vi "test - array in seperated but same session.vi"(8 "error in (no error)":errorcluster, 11 "TestCase in":refnum<class "labview-config-library.lvclass">) -> (0 "error out":errorcluster, 3 "TestCase out":refnum<class "labview-config-library.lvclass">)   [LabVIEW 2017, in "labview-config-library.lvclass"]
uses:
  labview-config-library.lvclass
  <vilib>/addons/_JKI Toolkits/VI Tester/TestCase.llb/TestCase.lvclass
  INI-Static-Variable-Support/LabVIEW-Config/LabVIEW-Config.lvclass
  INI-Static-Variable-Support/LabVIEW-Config/Read Array Key (Raw).vi
  C:/Program Files (x86)/National Instruments/LabVIEW 2017/vi.lib/addons/_JKI Toolkits/VI Tester/TestCase.llb/TestCase.lvclass
panel:
  out "appended array":bool[](array[boolean])
  out "text":string
  in  "Tab Control":enum32{"Page 1", "Page 2", "Page 3"}(tab)
  out "Section Names":string[](array[string])
  out "Key Names":string[](array[string])
  out "Array":string[](array[string])
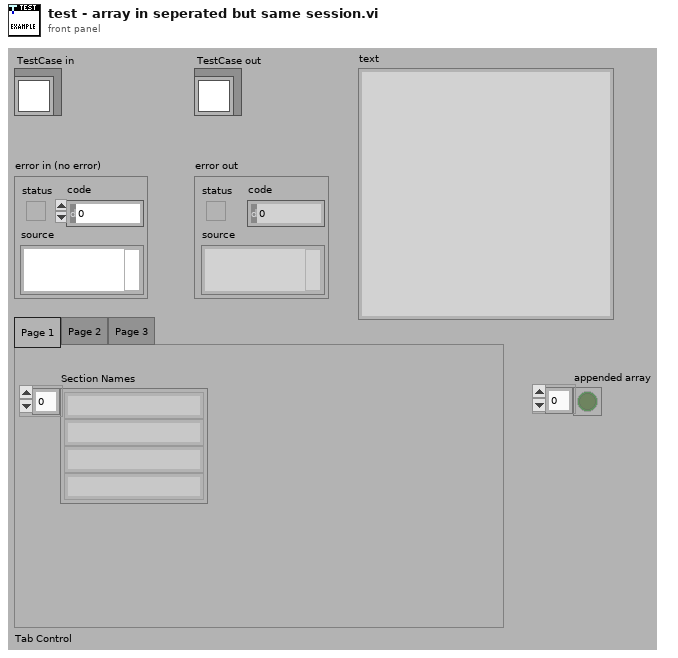
[diagram p1: front panel]
types:
  T1 = typedef "LabVIEW-Config.lvlib/LabVIEW-Config.lvclass/Config.ctl" = cluster{"Path":path, "Lines":string[], "Tokens":T2[], "Modified?":bool, "Cache":cluster{"Valid?":bool, "Key Information":T3[]}}
  T2 = typedef "LabVIEW-Config.lvlib/LabVIEW-Config.lvclass/LineToken.ctl" = enum8{"comment", "section", "key", "more"}
  T3 = typedef "LabVIEW-Config.lvlib/LabVIEW-Config.lvclass/KeyInfo.ctl" = cluster{"Key Indexes":cluster{"Indexes":i32[]}[], "Session Found?":bool, "Key found?":bool, "Session Index":i32}
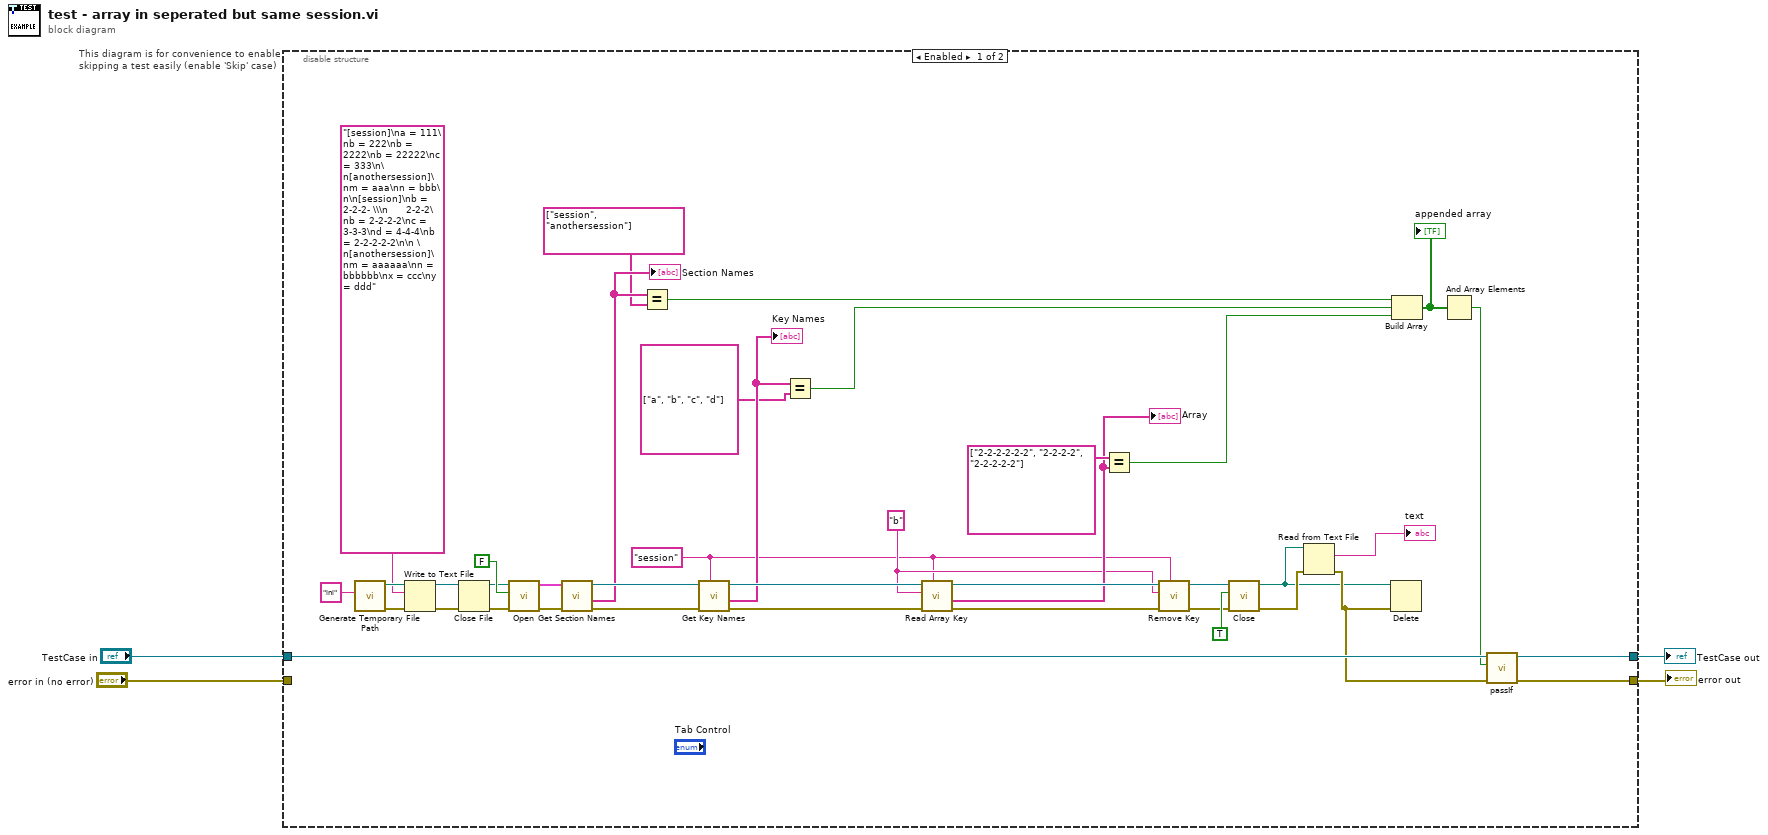
[diagram p0: block diagram]
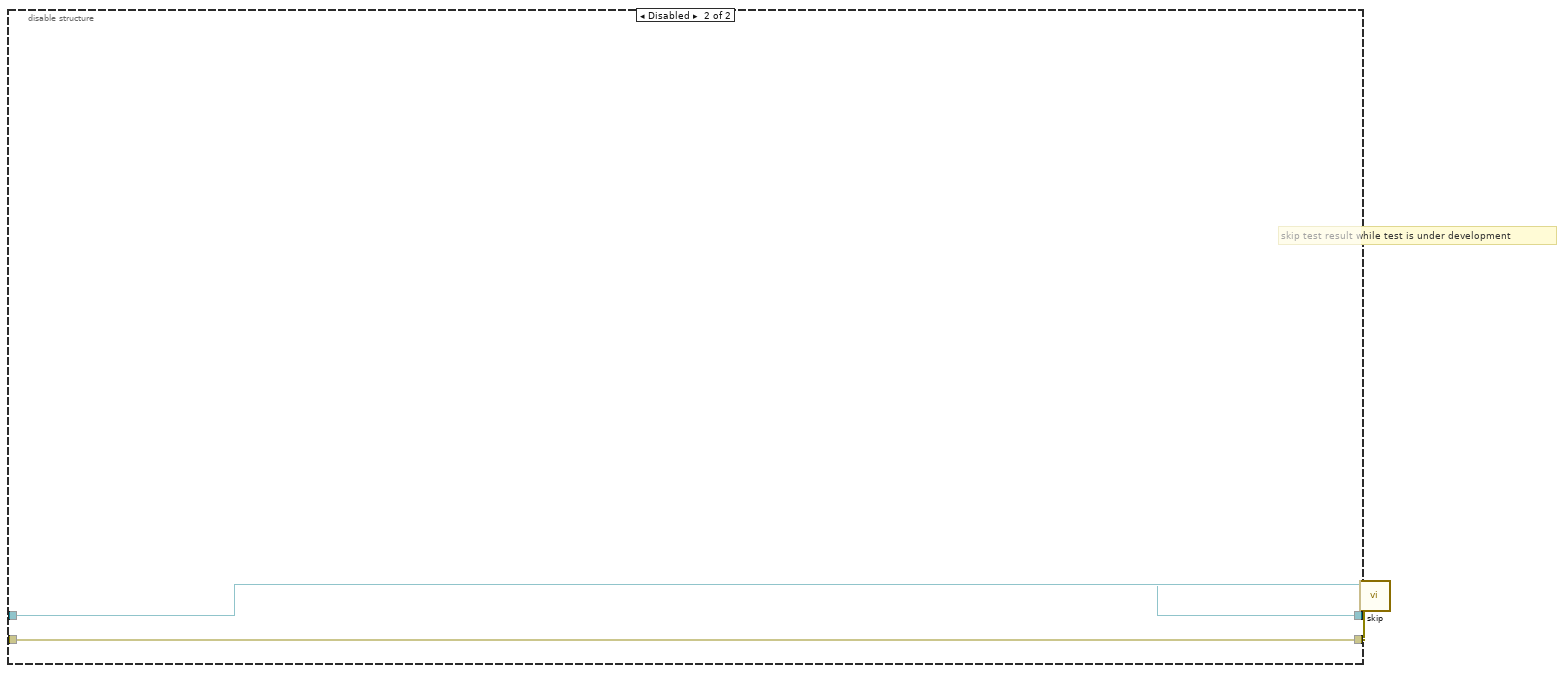
[diagram p2: hidden frame]
diagram:
  n1 = disable-structure "This diagram is for convenience to enable skipping a test easily (enable 'Skip' case)" shown="Enabled" {
    disable-tunnel: "TestCase in" -> [w44 w48]
    disable-tunnel: [w43 w46] -> w1
    disable-tunnel: [w42 w47] -> w3
    disable-tunnel: "error in (no error)" -> [_ w45]
    frame Enabled {
      w10 = "b" ("Section Name")
      w5 = "session" ("Section Name")
      # "Create temporary ini file"
      n2 = call <vilib>:"Generate Temporary File Path.vi"("Temporary File Extension (tmp)"="ini") -> ("error out"=w39:errorcluster, "Unique Temporary File Path"=w36:path)  [unwired: 9 in]
      n3 = Write to Text File(file (use dialog)=w36, text="[session]\na = 111\nb = 222\nb = 2222\nb = 22222\nc = 333\n\n[anothersession]\nm = aaa\nn = bbb\n\n[session]\nb = 2-2-2- \\\n      2-2-2\nb = 2-2-2-2\nc = 3-3-3\nd = 4-4-4\nb = 2-2-2-2-2\n\n \n[anothersession]\nm = aaaaaa\nn = bbbbbb\nx = ccc\ny = ddd", error in=w39) -> (refnum out=w35:refnum<file>, error out=w37:errorcluster)  [unwired: 1 in, 1 out]
      n4 = Close File(refnum=w35, error in=w37) -> (path=w32:path, error out=w33:errorcluster)
      n5 = call "Open.vi"("error in (no error)"=w33, "Create if not exists? (T)"=FALSE, "Path"=w32) -> ("error out"=w30:errorcluster, "Config"=w31:T1)  [unwired: 5 in, 2 out]
      n6 = call "Get Section Names.vi"("error in (no error)"=w30, "Config in"=w31) -> ("error out"=w26:errorcluster, "Section Names"=w25:string[], "Config out"=w27:refnum<class "LabVIEW-Config.lvclass">)  [unwired: 7 in]
      "Section Names" <- w25
      n7 = Equal?(x=w25, y=string[] ["session", "anothersession"]) -> (x = y?=w23:bool)
      n8 = call "Get Key Names.vi"("Section Name"=w5, "error in (no error)"=w26, "Config in"=w27) -> ("error out"=w29:errorcluster, "Key Names"=w21:string[], "Config out"=w28:refnum<class "LabVIEW-Config.lvclass">)  [unwired: 5 in, 1 out]
      "Key Names" <- w21
      n9 = Equal?(x=w21, y=string[] ["a", "b", "c", "d"] ("Key Names")) -> (x = y?=w20:bool)
      n10 = call-poly "Read Array Key.vi"("Section Name"=w5, "error in (no error)"=w29, "Key Name"=w10, "Config in"=w28) -> ("error out"=w16:errorcluster, "Content"=w11:string[], "Config out"=w17:refnum<class "LabVIEW-Config.lvclass">)  [unwired: 4 in, 1 out]
      "Array" <- w11
      n11 = Equal?(x=string[] ["2-2-2-2-2-2", "2-2-2-2", "2-2-2-2-2"] ("Key Names"), y=w11) -> (x = y?=w18:bool)
      n12 = call "Remove Key.vi"("Section Name"=w5, "error in (no error)"=w16, "Key Name"=w10, "Config in"=w17) -> ("error out"=w14:errorcluster, "Config out"=w15:refnum<class "LabVIEW-Config.lvclass">)  [unwired: 5 in, 1 out]
      n13 = call "Close.vi"("error in (no error)"=w14, "Write if modified? (T)"=TRUE, "Config"=w15) -> ("error out"=w9:errorcluster, "Path"=w7:path)  [unwired: 7 in]
      n14 = Read from Text File(file (use dialog)=w7, error in=w9) -> (text=→"text":string, error out=w8:errorcluster)  [unwired: 2 in, 2 out]
      n15 = Delete(path (use dialog)=w7, error in=w8) -> ()  [unwired: 3 in, 3 out]
      n16 = Build Array(w23, w20, w18) -> (w22:bool[])
      "appended array" <- w22
      n17 = And Array Elements(Boolean array=w22) -> (logical AND=w19:bool)
      n18 = call-dynamic "passIf.vi"("error in (no error)"=w8, "pass"=w19, "TestCase in"=w44) -> ("error out"=w42:errorcluster, "TestCase out"=w43:refnum<class "labview-config-library.lvclass">)  [unwired: 7 in]
    }
    frame Disabled {
      # "skip test result while test is under development"
      n19 = call <vilib>:"skip.vi"("error in (no error)"=w45, "TestCase in"=w48) -> ("error out"=w47:errorcluster, "TestCase out"=w46:refnum<class "labview-config-library.lvclass">)  [unwired: 8 in]
    }
  }
  "error out" <- w3
  "TestCase out" <- w1
